vi "Acquire_Temporal.vi"(8 "error in (no error)":errorcluster, 11 "FROG in":refnum<class "FROG.lvclass">) -> (0 "error out":errorcluster, 1 "String":string, 2 "frogTrace":T1, 3 "FROG out":refnum<class "FROG.lvclass">)   [LabVIEW 2020, in "FROG.lvclass"]
uses:
  FROG.lvclass
  IMAQ Image.ctl
  FROG.lvclass/FROG.ctl
  GUIcompressionCluster.ctl
  OnOffTypeDef.ctl
  Filter Error Codes (Array)__ogtk.vi
  CompressAndUpdate(Numeric).vi
  CompressAndUpdate(IMAQ Image).vi
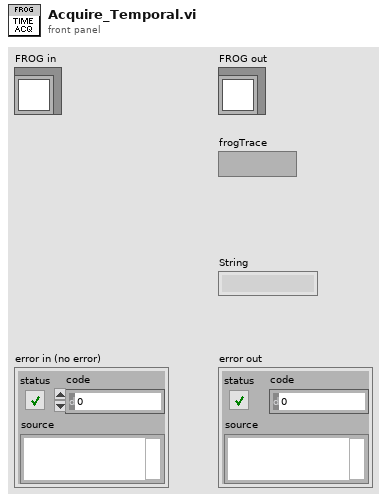
[diagram p1: front panel]
types:
  T1 = typedef "IMAQ Image.ctl" = refnum<image>
  T2 = typedef "GUIcompressionCluster.ctl" = cluster{"GUI8bit":T3, "GUICompression":T3, "CompressionQuality":i32}
  T3 = typedef "OnOffTypeDef.ctl" = enum16{"off", "on"}
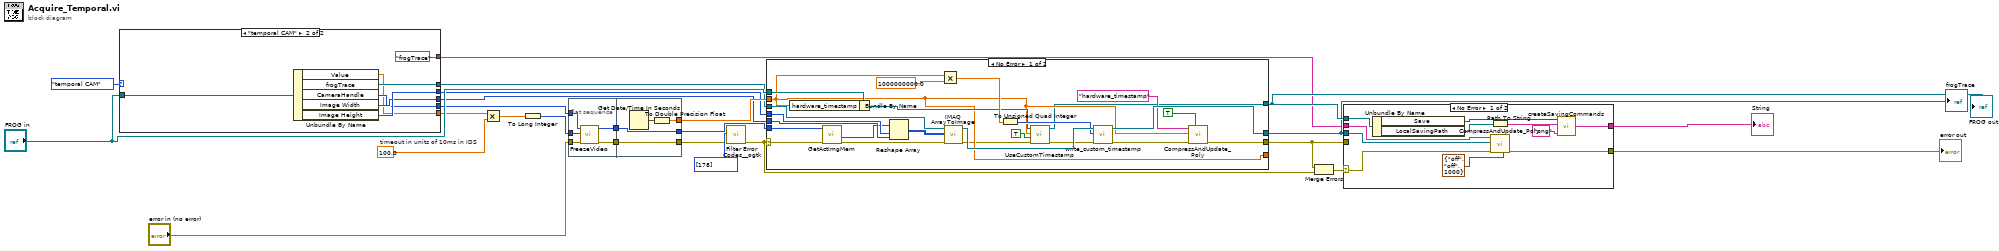
[diagram p0: block diagram]
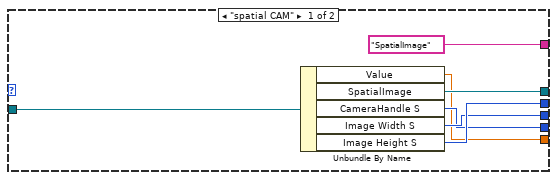
[diagram p2: hidden frame]
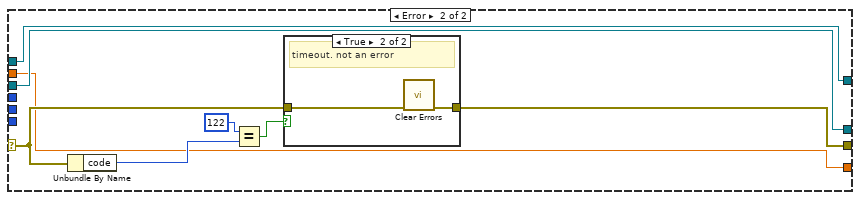
[diagram p4: hidden frame]
diagram:
  w6 = 100.0  # timeout in units of 10ms in IDS
  n1 = case shown="\"temporal CAM\"" enum16{"temporal CAM", "spatial CAM"}."temporal CAM" ("cameraselect") {
    tunnel: [w32 w39] -> w1
    tunnel: [w31 w38] -> w2
    tunnel: [w30 w37] -> w3
    tunnel: [w29 w36] -> w4
    tunnel: [w28 w35] -> w7
    tunnel: "FROG in" -> [w27 w34]
    tunnel: ["SpatialImage" ("command or variable name") "frogTrace" ("command or variable name")] -> w12
    frame "spatial CAM" {
      n2 = Unbundle By Name ("pressure read")(w27) -> ("Value"=w28:dbl, "SpatialImage"=w32:T1, "CameraHandle S"=w29:u32, "Image Width S"=w30:i32, "Image Height S"=w31:i32)
    }
    frame "temporal CAM" {
      n3 = Unbundle By Name ("pressure read")(w34) -> ("Value"=w35:dbl, "frogTrace"=w39:T1, "CameraHandle"=w36:u32, "Image Width"=w37:i32, "Image Height"=w38:i32)
    }
  }
  n4 = Multiply(x=w7, y=w6) -> (x*y=w8:dbl)
  n5 = To Long Integer(number=w8) -> (32bit integer=w5:i32)
  n6 = flat-sequence {
    tunnel: w4 -> [w44]
    tunnel: w5 -> [w43]
    tunnel: "error in (no error)" -> [w41]
    tunnel: [w42] -> w25
    tunnel: [w40] -> w24
    tunnel: [w47] -> w17
    tunnel: [w48] -> w9
    tunnel: w25 -> [w48]
    tunnel: w24 -> [w47]
    tunnel: [w45] -> w22
    frame #0 {
      n7 = call "FreezeVideo.vi"("error in"=w41, "Wait"=w43, "Camera Handle In"=w44) -> ("error out"=w40:errorcluster, "Camera Handle Out"=w42:u32)  [unwired: 7 out]
    }
    frame #1 {
      n8 = Get Date/Time In Seconds() -> (seconds since 1Jan1904=w46:timestamp)
      n9 = To Double Precision Float(number=w46) -> (double precision float=w45:dbl)
    }
  }
  n10 = call-poly "Filter Error Codes__ogtk.vi"("Error In"=w17, "Error Codes to Filter"=i32[] [178]) -> ("Error Out"=w18:errorcluster)  [unwired: 7 in, 2 out]
  n11 = case shown="No Error" w18 {
    selector: w18 -> [w65 w75]
    tunnel: w1 -> [w72 w77]
    tunnel: w3 -> [w71 _]
    tunnel: w2 -> [w70 _]
    tunnel: w9 -> [w68 _]
    tunnel: [w55 w76] -> w11
    tunnel: [w63 w77] -> w19
    tunnel: "FROG in" -> [w59 w74]
    tunnel: [w51 w74] -> w20
    tunnel: w22 -> [w53 w73]
    tunnel: [w53 w73] -> _
    frame No Error {
      n12 = Bundle By Name(cluster=w59, "hardware_timestamp"=w53) -> (w54:refnum<class "FROG.lvclass">)
      n13 = call "GetActImgMem.vi"("error in"=w65, "Camera Handle In"=w68) -> ("error out"=w69:errorcluster, "Image Memory Out"=w67:u8[])  [unwired: 8 out]
      n14 = Reshape Array(w67, w70, w71) -> (w66:u8[][])
      n15 = Multiply(x=w53, y=1000000000.0) -> (x*y=w61:dbl)
      n16 = call "IMAQ ArrayToImage"("error in (no error)"=w69, "Image Pixels (U8)"=w66, "Image"=w72) -> ("error out"=w50:errorcluster, "Image Out"=w64:T1)  [unwired: 7 in]
      n17 = To Unsigned Quad Integer(1:w61) -> (0:w60:u64)
      n18 = call-dynamic "UseCustomTimestamp.vi"("error in (no error)"=w50, "AcqSuccess"=TRUE, "CustomTimeStamp"=w53, "BaseDriver in"=w54) -> ("error out"=w49:errorcluster, "BaseDriver out"=w51:refnum<class "FROG.lvclass">)  [unwired: 6 in]
      n19 = call "write_custom_timestamp.vi"("error in (no error)"=w49, "timestamp (ns)"=w60, "Refnum in"=w64) -> ("error out"=w56:errorcluster, "Refnum out"=w63:T1)  [unwired: 7 in]
      n20 = call-poly "CompressAndUpdate_Poly.vi"("force CVT update (false)"=TRUE, "error in"=w56, "Numeric"=w53, "command or variable name"="hardware_timestamp") -> ("error out"=w55:errorcluster)  [unwired: 7 in]
    }
    frame Error {
      n21 = Unbundle By Name(w75) -> ("code"=w80:i32)
      n22 = Equal?(x=122, y=w80) -> (x = y?=w78:bool)
      n23 = case shown="True" w78 {
        tunnel: w75 -> [w81 w83]
        tunnel: [w81 w82] -> w76
        frame False {
        }
        frame True {
          # "timeout. not an error"
          n24 = call "Clear Errors.vi"("error in (no error)"=w83) -> ("error out"=w82:errorcluster)  [unwired: 5 in, 1 out]
        }
      }
    }
  }
  "FROG out" <- w20
  "frogTrace" <- w19
  n25 = Merge Errors(w11, w18) -> (w10:errorcluster)
  n26 = case shown="No Error" w10 {
    selector: w10 -> [w91 _]
    tunnel: [w92 w95] -> w14
    tunnel: w19 -> [w93 _]
    tunnel: w11 -> [_ w95]
    tunnel: w12 -> [w90 _]
    tunnel: [w87 _] -> w15
    tunnel: w20 -> [w84 _]
    frame No Error {
      n27 = Unbundle By Name ("pressure read")(w84) -> ("Save"=w86:T3, "LocalSavingPath"=w85:path)
      n28 = Path To String(path=w85) -> (string=w89:string)
      n29 = call-poly "CompressAndUpdate_Poly.vi"("GUICompression"=T2 {"GUI8bit"=enum."off", "GUICompression"=enum."off", "CompressionQuality"=1000}, "error in"=w91, "IMAQ Image"=w93, "command or variable name"=w90) -> ("error out"=w92:errorcluster)  [unwired: 7 in]
      n30 = call "createSavingCommands.vi"("extension"="png", "Saving Path (local)"=w89, "Save"=w86) -> ("String"=w87:string)  [unwired: 1 in]
    }
    frame Error {
    }
  }
  "String" <- w15
  "error out" <- w14
